vi "Annotations Tip Strip Ref FGV.vi"(1 "Action(GET)":T2(ring), 7 "References in":T1, 11 "error in (no error)":errorcluster) -> (8 "References Out":T1, 15 "error out":errorcluster)   [LabVIEW 2011]
uses:
  Annotations Tip Strip FGV_cluster.ctl
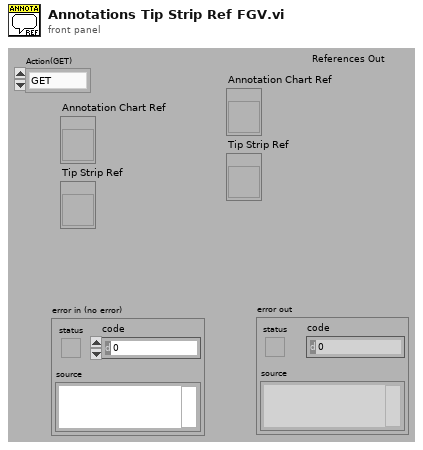
[diagram p1: front panel]
types:
  T1 = typedef "Annotations Tip Strip FGV_cluster.ctl" = cluster{"Annotation Chart Ref":refnum<vi>, "Tip Strip Ref":refnum<vi>}
  T2 = enum16{"GET", "SET", "Get from Ini", "Put in Ini"}
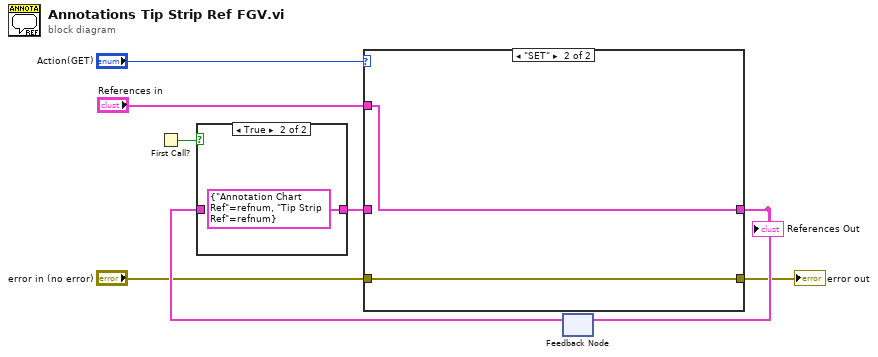
[diagram p0: block diagram]
diagram:
  n1 = First Call?() -> (First Call?: T/F=w7:bool)
  n2 = feedback #1() -> (w8:T1)  [unwired: 1 in]
  n3 = case shown="True" w7 {
    tunnel: w8 -> [w9 _]
    tunnel: [w9 T1 {"Annotation Chart Ref"=refnum, "Tip Strip Ref"=refnum} ("User ID in")] -> w5
    frame False {
    }
    frame True {
    }
  }
  n4 = case shown="\"SET\"" "Action(GET)" {
    tunnel: [w12 w14] -> w6
    tunnel: w5 -> [w12 _]
    tunnel: "References in" -> [_ w14]
    tunnel: "error in (no error)" -> [w11 w13]
    tunnel: [w11 w13] -> w1
    frame "GET", Default {
    }
    frame "SET" {
    }
  }
  "error out" <- w1
  "References Out" <- w6
  n5 = feedback-in #1(w6) -> ()
